vi "flow_rate_sensor_model.vi"(10 "input(A)":dbl) -> (2 "output(LPM)":dbl)   [LabVIEW 2020]
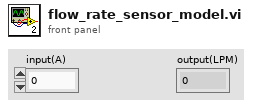
[diagram p1: front panel]
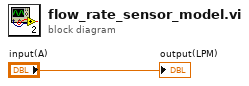
[diagram p0: block diagram]
diagram:
  "output(LPM)" <- "input(A)"
